vi "Get Output Values.vi"(6 "Last request":bool, 8 "error in (no error)":errorcluster, 10 "Number of points":i32, 11 "Spectrum Recorder in":refnum<class "Spectrum Recorder too.lvclass">) -> (0 "error out":errorcluster, 1 "Reset":bool, 2 "Output values":dbl[](array[numeric]), 3 "Spectrum Recorder out":refnum<class "Spectrum Recorder too.lvclass">)   [LabVIEW 2016, in "Spectrum Recorder too.lvclass"]
uses:
  Spectrum Recorder too.lvclass
  C:/github/LabActor/Instrument Actor/Instrument Actor.lvclass
  Spectrum Recorder too.lvclass/Spectrum Recorder too.ctl
  Read Spectrum Recorder Configuration.vi
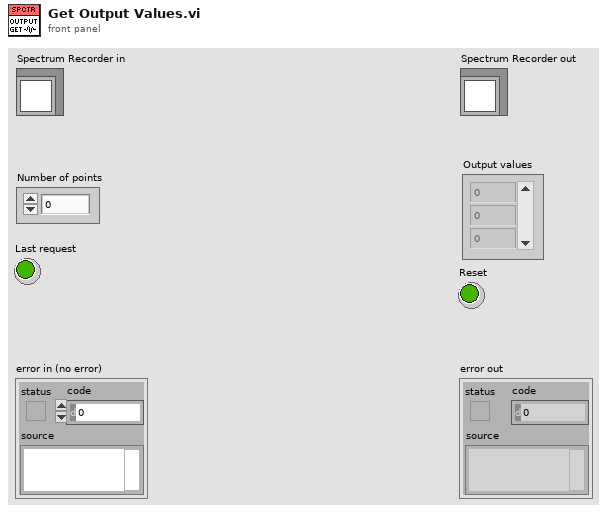
[diagram p1: front panel]
types:
  T1 = typedef "Spectrum Configuration.ctl" = cluster{"Start frequency":dbl, "End frequency":dbl, "Coarse step":dbl, "Step duration":dbl, "Red Pitaya address":string, "Open plot \non start":bool, "Fine region centers":dbl[], "Regions width":dbl, "Fine step":dbl, "Pause between scans":dbl, "Clear rgs on start":bool, "Output amplitude":dbl}
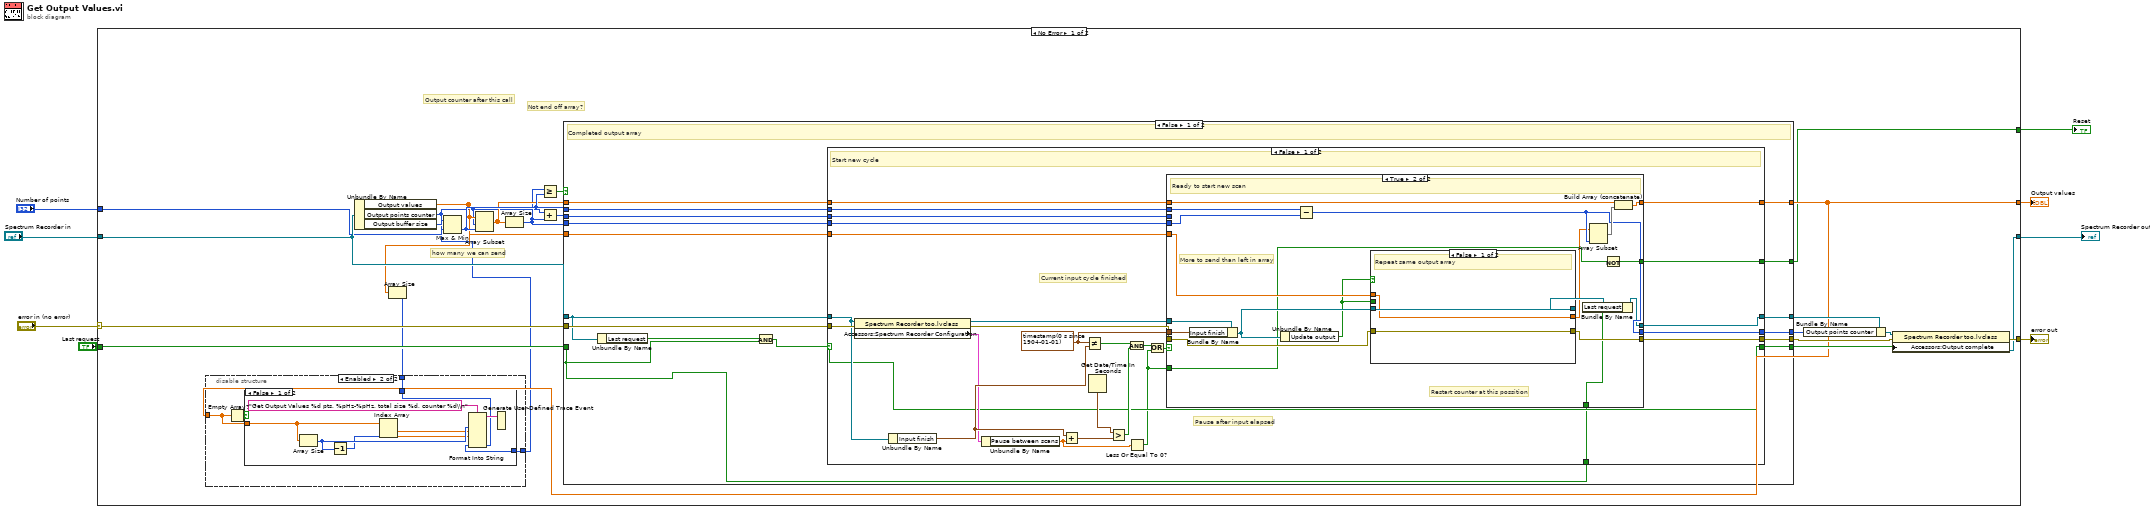
[diagram p0: block diagram]
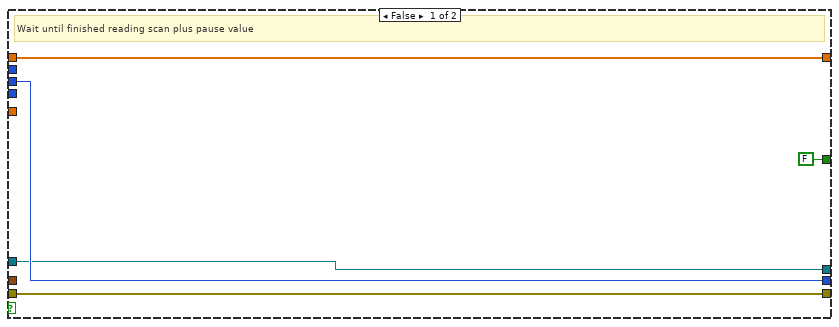
[diagram p4: hidden frame]
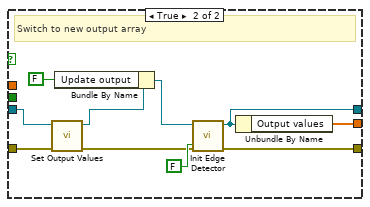
[diagram p5: hidden frame]
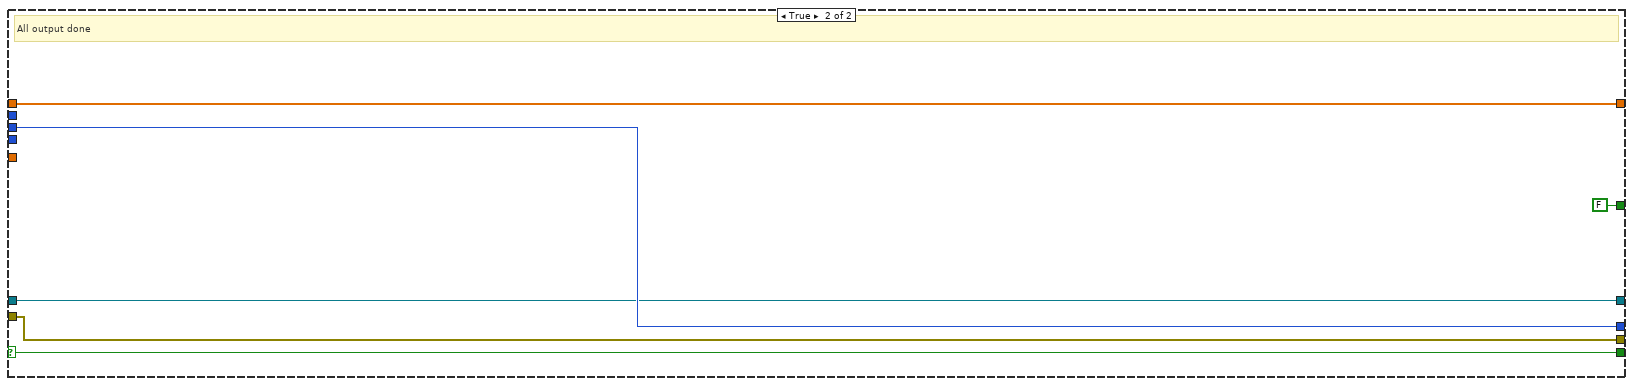
[diagram p6: hidden frame]
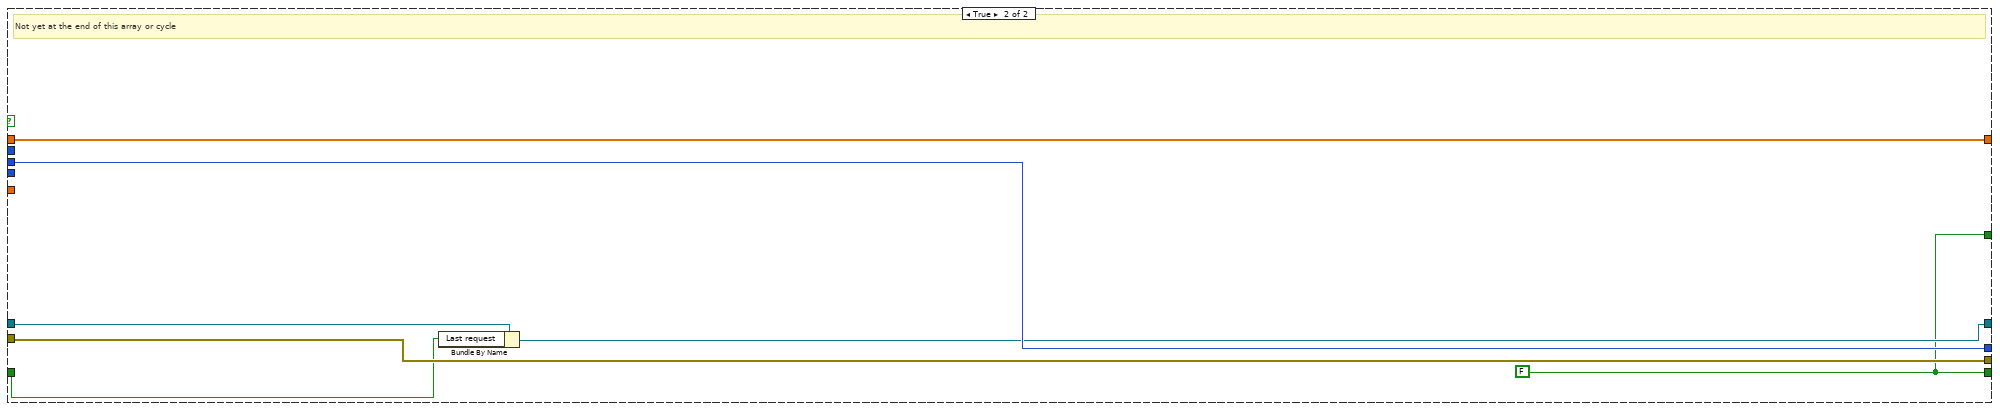
[diagram p7: hidden frame]
diagram:
  n1 = case shown="No Error" "error in (no error)" {
    selector: "error in (no error)" -> [w15 w138]
    tunnel: [w30 w138] -> w7
    tunnel: [w28 w137] -> w5
    tunnel: "Spectrum Recorder in" -> [w25 w137]
    tunnel: "Number of points" -> [w19 _]
    tunnel: [w13 _] -> w3
    tunnel: "Last request" -> [w26 _]
    tunnel: [w9 _] -> w1
    frame No Error {
      # "Not end off array?"
      # "Output counter after this call"
      # "how many we can send"
      n2 = Unbundle By Name(w25) -> ("Output values"=w12:dbl[], "Output points counter"=w10:i32, "Output buffer size"=w18:i32)
      n3 = Array Size(array=w12) -> (size(s)=w11:i32)
      n4 = Max & Min(x=w18, y=w19) -> (min(x,y)=w24:i32)  [unwired: 1 out]
      n5 = Array Subset(array=w12, index=w10, length=w24) -> (w22:dbl[])
      n6 = Array Size(array=w22) -> (size(s)=w17:i32)
      n7 = Greater Or Equal?(x=w17, y=w24) -> (x >= y?=w27:bool)
      n8 = Add(x=w10, y=w17) -> (x+y=w21:i32)
      n9 = case shown="False" w27 {
        tunnel: w12 -> [w59 _]
        tunnel: w21 -> [w53 w135]
        tunnel: w24 -> [w50 _]
        tunnel: w26 -> [w45 w131]
        tunnel: w25 -> [w48 w134]
        tunnel: [w57 w136] -> w13
        tunnel: w22 -> [w58 w136]
        tunnel: [w46 w130] -> w23
        tunnel: [w56 w135] -> w14
        tunnel: [w55 w132] -> w20
        tunnel: w17 -> [w54 _]
        tunnel: [w52 w133] -> w16
        tunnel: w15 -> [w51 w133]
        tunnel: [w44 w130] -> w9
        frame False {
          # "Completed output array"
          n10 = Unbundle By Name(w48) -> ("Last request"=w47:bool)
          n11 = And(x=w47, y=w45) -> (x .and. y?=w49:bool)
          n12 = case shown="False" w49 {
            selector: w49 -> [w63 w129]
            tunnel: w48 -> [w67 w127]
            tunnel: w59 -> [w86 _]
            tunnel: w58 -> [w85 w126]
            tunnel: w53 -> [w65 w128]
            tunnel: [w84 w126] -> w57
            tunnel: [w63 w129] -> w46
            tunnel: [w83 w128] -> w56
            tunnel: [w80 w127] -> w55
            tunnel: w54 -> [w82 _]
            tunnel: [w79 w125] -> w52
            tunnel: w51 -> [w78 w125]
            tunnel: w50 -> [w81 _]
            tunnel: w45 -> [w62 _]
            tunnel: [w60 FALSE] -> w44
            frame False {
              w64 = timestamp(0 s since 1904-01-01)
              # "Pause after input elapsed"
              # "Current input cycle finished"
              # "Start new cycle"
              n13 = property class="Spectrum Recorder too.lvclass"(reference=w67, error in=w78) -> (reference out=w66:refnum<class "Spectrum Recorder too.lvclass">, error out=w69:errorcluster, "Accessors:Spectrum Recorder Configuration"=w70:T1)
              n14 = Unbundle By Name(w67) -> ("Input finish"=w74:timestamp)
              n15 = Unbundle By Name(w70) -> ("Pause between scans"=w71:dbl)
              n16 = Add(x=w74, y=w71) -> (x+y=w73:timestamp)
              n17 = Not Equal?(x=w64, y=w74) -> (x != y?=w77:bool)
              n18 = Get Date/Time In Seconds() -> (seconds since 1Jan1904=w72:timestamp)
              n19 = Greater?(x=w72, y=w73) -> (0:w76:bool)
              n20 = And(x=w77, y=w76) -> (x .and. y?=w75:bool)
              n21 = Less Or Equal To 0?(x=w71) -> (x <= 0?=w61:bool)
              n22 = Or(x=w75, y=w61) -> (x .or. y?=w68:bool)
              n23 = case shown="True" w68 {
                tunnel: w66 -> [w89 w110]
                tunnel: w86 -> [_ w109]
                tunnel: w85 -> [w91 w108]
                tunnel: [w91 w106] -> w84
                tunnel: [w90 w105] -> w83
                tunnel: w82 -> [_ w104]
                tunnel: w69 -> [w88 w103]
                tunnel: w81 -> [_ w102]
                tunnel: [w89 w96] -> w80
                tunnel: [w88 w100] -> w79
                tunnel: w65 -> [w90 _]
                tunnel: w64 -> [_ w97]
                tunnel: w62 -> [_ w95]
                tunnel: [FALSE w92] -> w60
                tunnel: w61 -> [_ w93]
                frame False {
                  # "Wait until finished reading scan plus pause value"
                }
                frame True {
                  # "Restart counter at this possition"
                  # "More to send than left in array"
                  # "Ready to start new scan"
                  n24 = Bundle By Name(cluster=w110, "Input finish"=w97) -> (w98:refnum<class "Spectrum Recorder too.lvclass">)
                  n25 = Unbundle By Name(w98) -> ("Update output"=w94:bool)
                  n26 = Subtract(x=w102, y=w104) -> (x-y=w105:i32)
                  n27 = case shown="False" w94 {
                    tunnel: w98 -> [w113 w115]
                    tunnel: w94 -> [_ _]
                    tunnel: [w113 w117] -> w101
                    tunnel: [w112 w116] -> w99
                    tunnel: w109 -> [w112 _]
                    tunnel: [w111 w122] -> w100
                    tunnel: w103 -> [w111 w119]
                    frame False {
                      # "Repeat same output array"
                    }
                    frame True {
                      # "Switch to new output array"
                      n28 = call-dynamic "Set Output Values.vi"("error in (no error)"=w119, "Spectrum Recorder in"=w115) -> ("error out"=w118:errorcluster, "Spectrum Recorder out"=w114:refnum<class "Spectrum Recorder too.lvclass">)  [unwired: 8 in]
                      n29 = Bundle By Name(cluster=w114, "Update output"=FALSE) -> (w123:refnum<class "Spectrum Recorder too.lvclass">)
                      n30 = call-dynamic "Init Edge Detector.vi"("Unsee last word"=FALSE, "error in (no error)"=w118, "Spectrum Recorder too in"=w123) -> ("error out"=w122:errorcluster, "Spectrum Recorder too out"=w117:refnum<class "Spectrum Recorder too.lvclass">)  [unwired: 7 in]
                      n31 = Unbundle By Name(w117) -> ("Output values"=w116:dbl[])
                    }
                  }
                  n32 = Bundle By Name(cluster=w101, "Last request"=w95) -> (w96:refnum<class "Spectrum Recorder too.lvclass">)
                  n33 = Array Subset(array=w99, length=w105) -> (w107:dbl[])  [unwired: 1 in]
                  n34 = Not(x=w93) -> (.not. x?=w92:bool)
                  n35 = Build Array (concatenate)(w108, w107) -> (w106:dbl[])
                }
              }
            }
            frame True {
              # "All output done"
            }
          }
        }
        frame True {
          w130 = FALSE
          # "Not yet at the end of this array or cycle"
          n36 = Bundle By Name(cluster=w134, "Last request"=w131) -> (w132:refnum<class "Spectrum Recorder too.lvclass">)
        }
      }
      n37 = disable-structure shown="Enabled" {
        disable-tunnel: w13 -> [_ w33]
        disable-tunnel: w11 -> [_ w32]
        disable-tunnel: w10 -> [_ w31]
        frame Disabled {
        }
        frame Enabled {
          n38 = Empty Array?(array=w33) -> (empty?=w34:bool)
          n39 = case shown="False" w34 {
            tunnel: w33 -> [w42 _]
            tunnel: w32 -> [w36 _]
            tunnel: w31 -> [w35 _]
            frame False {
              n40 = Array Size(array=w42) -> (size(s)=w41:i32)
              n41 = Decrement(x=w41) -> (x-1=w40:i32)
              n42 = Index Array(array=w42, index #2=w40) -> (element #1=w39:dbl, element #2=w38:dbl)  [unwired: 1 in]
              n43 = Format Into String(format string="Get Output Values %d pts, %pHz-%pHz, total size %d, counter %d\\n", w41, w39, w38, w36, w35) -> (resulting string=w37:string)  [unwired: 2 in, 1 out]
              n44 = Generate User-Defined Trace Event(2:w37) -> ()  [unwired: 1 in]
            }
            frame True {
            }
          }
        }
      }
      n45 = Bundle By Name(cluster=w20, "Output points counter"=w14) -> (w29:refnum<class "Spectrum Recorder too.lvclass">)
      n46 = property class="Spectrum Recorder too.lvclass"(reference=w29, error in=w16, "Accessors:Output complete"=w23) -> (reference out=w28:refnum<class "Spectrum Recorder too.lvclass">, error out=w30:errorcluster)
    }
    frame Error {
    }
  }
  "error out" <- w7
  "Spectrum Recorder out" <- w5
  "Output values" <- w3
  "Reset" <- w1
